vi "list available jl functions.vi"(8 "error in (no error)":errorcluster) -> (0 "error out":errorcluster, 1 "Jl Server state out":T1, 3 "ext_fns":string[](array[string]), 4 "detailed error info":T2, 5 "return code":u8, 7 "timeout?":bool)   [LabVIEW 2018, in "LV-0mq-Julia_roundtrip-lib.lvlib"]
doc: "List function available on Server."
uses:
  LV-0mq-Julia_roundtrip-lib.lvlib
  detailed error info.ctl
  StackFrame.ctl
  Server or client state.ctl
  318091ce-7b2e-4b52-a944-14c6363efdda.vi
  318091ce-7b2e-4b52-a944-14c6363efdda.vi/1032d8ef-ffdb-4eb5-8ce9-9cb9272a0550.vi
  318091ce-7b2e-4b52-a944-14c6363efdda.vi/1032d8ef-ffdb-4eb5-8ce9-9cb9272a0550.vi/c7ea1634-287b-4fd5-b233-0d5794ac535b.vi
  318091ce-7b2e-4b52-a944-14c6363efdda.vi/1032d8ef-ffdb-4eb5-8ce9-9cb9272a0550.vi/5ff2acd9-9f87-4932-af06-d8cc5dccd708.vi
  318091ce-7b2e-4b52-a944-14c6363efdda.vi/1032d8ef-ffdb-4eb5-8ce9-9cb9272a0550.vi/6d0d8ebb-cb2f-4243-996d-931c69cf3a45.vi
  check ID validity.vi
  bindata_descr to JSON.vi
  check cluster field names.vi
  concat JSON.vi
  build request.vi
  REQ full lifecycle.vi
  Parse server response.vi
  log jl exceptions.vi
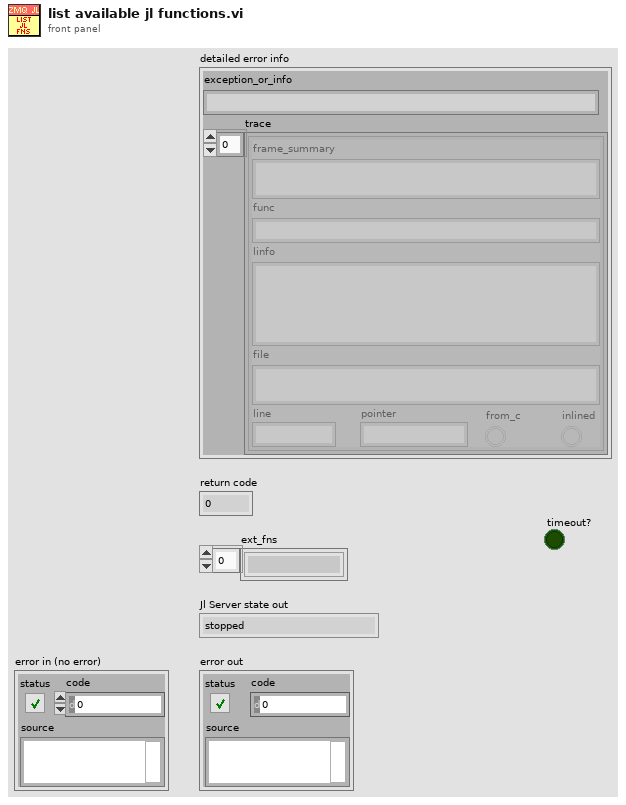
[diagram p1: front panel]
types:
  T1 = typedef "LV-0mq-Julia_roundtrip-lib.lvlib/Server or client state.ctl" = enum16{"stopped", "running", "unknown"}
  T2 = typedef "LV-0mq-Julia_roundtrip-lib.lvlib/detailed error info.ctl" = cluster{"exception_or_info":string, "trace":T3[]}
  T3 = typedef "LV-0mq-Julia_roundtrip-lib.lvlib/StackFrame.ctl" = cluster{"frame_summary":string, "func":string, "linfo":string, "file":string, "line":i32, "pointer":u64, "from_c":bool, "inlined":bool}
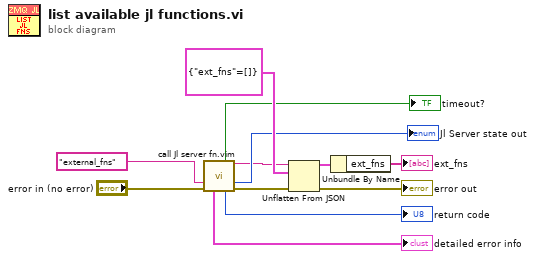
[diagram p0: block diagram]
diagram:
  n1 = call "call Jl server fn.vim"("fun2call"="external_fns", "error in (no error)"="error in (no error)") -> ("timeout?"=→"timeout?":bool, "JSON received"=w2:string, "Jl Server state out"=→"Jl Server state out":T1, "detailed error info"=→"detailed error info":T2, "return code"=→"return code":u8, "error out"=w3:errorcluster)  [unwired: 7 in, 1 out]
  n2 = Unflatten From JSON(JSON string=w2, type and defaults=cluster{"ext_fns":string[]} {"ext_fns"=[]}, error in (no error)=w3) -> (value=w11:cluster{"ext_fns":string[]}, error out=→"error out":errorcluster)  [unwired: 4 in]
  n3 = Unbundle By Name(w11) -> ("ext_fns"=→"ext_fns":string[])
